vi "FinalProjectofCSE360.vi"() -> ()   [LabVIEW 2020]
panel:
  out "VO2 (mL/kg.min)":dbl(slide) scale=0.0..2000.0
  out "Battery Status":dbl(slide) scale=0.0..100.0
  out "Heart Rate (bpm)":dbl(knob) scale=0.0..150.0
  in  "VISA resource name":refnum<visa-resource-name>
  in  "Table Control":string[][](table)
  out "Speed":dbl(graph)
  out "Heart Rate":dbl(graph)
  out "Speed (RPM)":dbl(knob) scale=0.0..100.0
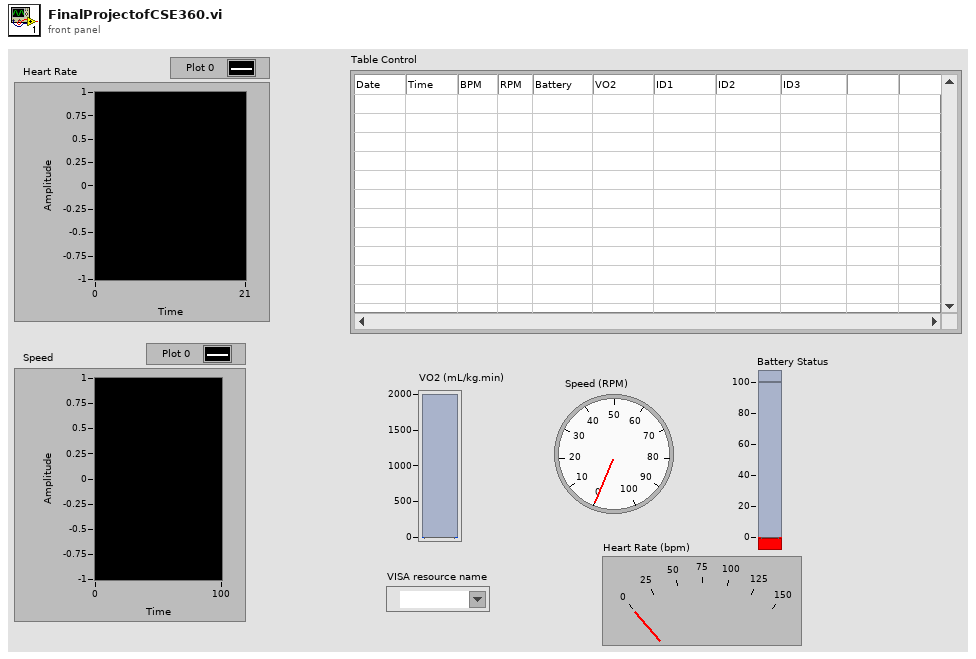
[diagram p1: front panel]
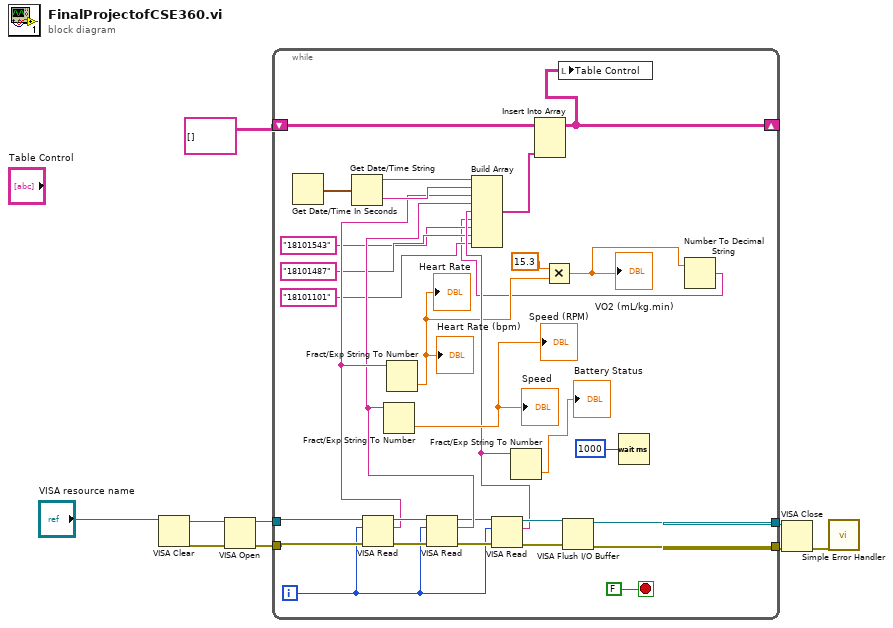
[diagram p0: block diagram]
diagram:
  n1 = VISA Clear(VISA resource name="VISA resource name") -> (VISA resource name out=w8:refnum<visa-resource-name>, error out=w7:errorcluster)  [unwired: 1 in]
  n2 = VISA Open(error in (no error)=w7, VISA resource name=w8) -> (VISA resource name=w6:refnum<visa-resource-name>, error out=w5:errorcluster)  [unwired: 3 in]
  n3 = while {
    tunnel: w6 -> [w40]
    tunnel: w5 -> [w39]
    tunnel: [w36] -> w3
    tunnel: [w35] -> w2
    shift-right: [w24] -> _
    shift-left: string[][] [] -> [w33]
    i -> [w21]
    stop <- FALSE stop-if-true
    n4 = Get Date/Time In Seconds() -> (seconds since 1Jan1904=w31:timestamp)
    n5 = Get Date/Time String(seconds (now)=w31) -> (date string=w30:string, time string=w29:string)  [unwired: 2 in]
    n6 = VISA Read(VISA resource name=w40, byte count=w21, error in (no error)=w39) -> (VISA resource name out=w38:refnum<visa-resource-name>, read buffer=w28:string, error out=w37:errorcluster)  [unwired: 1 out]
    n7 = Fract/Exp String To Number(string=w28) -> (number=w16:dbl)  [unwired: 3 in, 1 out]
    "Heart Rate" <- w16
    "Heart Rate (bpm)" <- w16
    n8 = VISA Read(VISA resource name=w38, byte count=w21, error in (no error)=w37) -> (VISA resource name out=w23:refnum<visa-resource-name>, read buffer=w27:string, error out=w22:errorcluster)  [unwired: 1 out]
    n9 = Fract/Exp String To Number(string=w27) -> (number=→"Speed (RPM)" →"Speed":dbl)  [unwired: 3 in, 1 out]
    n10 = VISA Read(VISA resource name=w23, byte count=w21, error in (no error)=w22) -> (VISA resource name out=w20:refnum<visa-resource-name>, read buffer=w18:string, error out=w19:errorcluster)  [unwired: 1 out]
    n11 = Fract/Exp String To Number(string=w18) -> (number=→"Battery Status":dbl)  [unwired: 3 in, 1 out]
    n12 = Multiply(x=15.3, y=w16) -> (x*y=w11:dbl)
    "VO2 (mL/kg.min)" <- w11
    n13 = VISA Flush I/O Buffer(VISA resource name=w20, error in (no error)=w19) -> (VISA resource name out=w36:refnum<visa-resource-name>, error out=w35:errorcluster)  [unwired: 1 in]
    n14 = Wait (ms)(milliseconds to wait=u32 1000) -> ()  [unwired: 1 out]
    n15 = Number To Decimal String(number=w11) -> (decimal integer string=w10:string)  [unwired: 1 in]
    n16 = Build Array(w30, w29, w28, w27, w18, w10, "18101543" ("element"), "18101487" ("element"), "18101101" ("element")) -> (w25:string[])
    n17 = Insert Into Array(array=w33, new element=w25) -> (w24:string[][])  [unwired: 2 in]
    n18 = local write "Table Control"(w24) -> ()
  }
  n19 = VISA Close(VISA resource name=w3, error in (no error)=w2) -> (error out=w9:errorcluster)
  n20 = call <vilib>:"Simple Error Handler.vi"("error in (no error)"=w9) -> ()  [unwired: 4 in, 5 out]
